vi "DEMO.vi"() -> ()   [LabVIEW 2013]
uses:
  Tag Data.lvclass
  Method/Add DBL to HashTable.vi
  Method/Get DBL Value from HashTable.vi
panel:
  out "Value":dbl
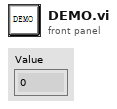
[diagram p1: front panel]
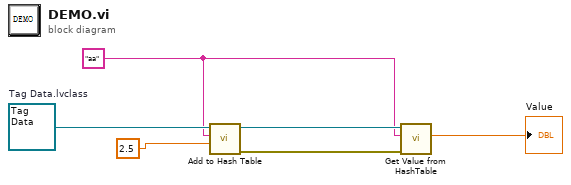
[diagram p0: block diagram]
diagram:
  w2 = "aa" ("Name")
  w6 = refnum<class "Tag Data.lvclass"> refnum  # Tag Data.lvclass
  n1 = call-poly "Add to Hash Table.vi"("Value"=2.5, "Name"=w2, "Contstant Base 输入"=w6) -> ("error out"=w4:errorcluster, "Contstant Base 输出"=w3:refnum<class "Tag Data.lvclass">)  [unwired: 7 in]
  n2 = call-poly "Get Value from HashTable.vi"("error in (no error)"=w4, "Name"=w2, "Contstant Base 输入"=w3) -> ("Value"=→"Value":dbl)  [unwired: 6 in, 2 out]
